vi "Add TypeDef to Cluster.vi"(5 "isArray (F)":bool, 7 "TypeDef path":path, 8 "error in (no error)":errorcluster, 10 "Message Element Name":string, 11 "Owning cluster ref in":refnum<vi>) -> (0 "error out":errorcluster, 2 "Control ref out":refnum<vi>, 3 "Owning cluster ref out":refnum<vi>)   [LabVIEW 2019, in "gRPC Scripting Tools.lvlib"]
uses:
  gRPC Scripting Tools.lvlib
  <vilib>/Utility/miscctls.llb/LVPointTypeDef.ctl
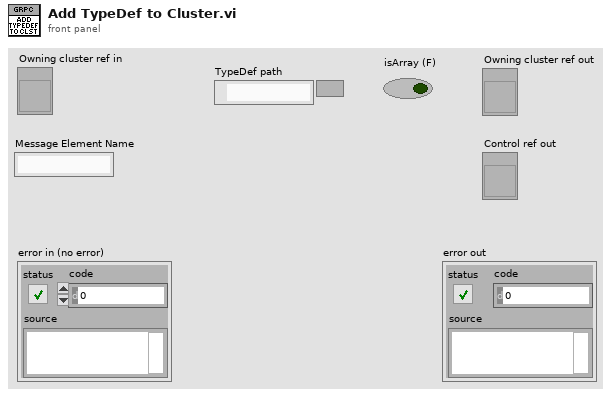
[diagram p1: front panel]
types:
  T1 = typedef "LVPointTypeDef.ctl" = cluster{"Horizontal":i16, "Vertical":i16}
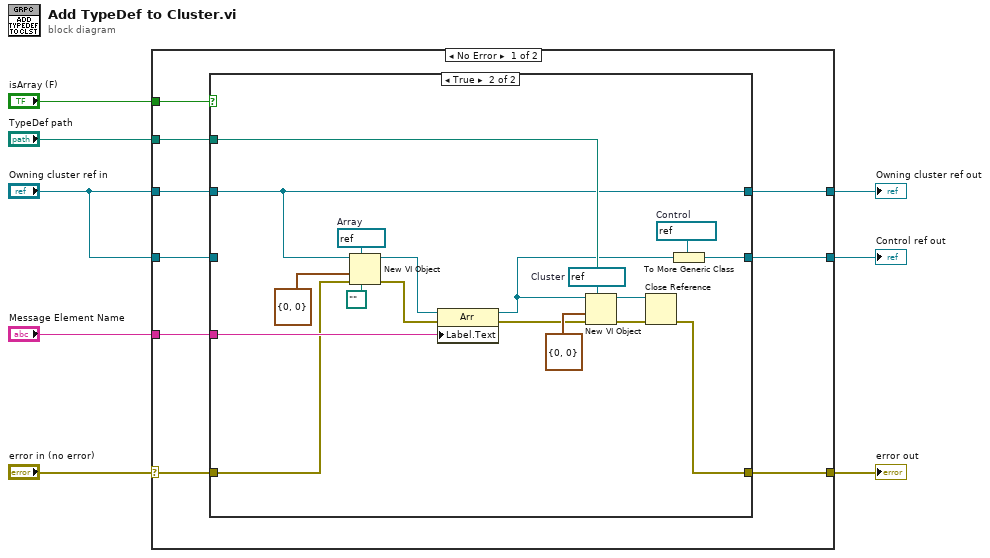
[diagram p0: block diagram]
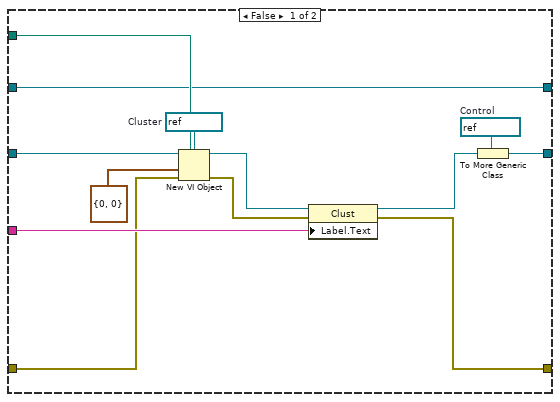
[diagram p2: hidden frame]
diagram:
  n1 = case shown="No Error" "error in (no error)" {
    selector: "error in (no error)" -> [w14 w50]
    tunnel: [w13 w50] -> w8
    tunnel: "TypeDef path" -> [w17 _]
    tunnel: "Owning cluster ref in" -> [w16 _]
    tunnel: "Message Element Name" -> [w15 _]
    tunnel: [w12 _] -> w1
    tunnel: "Owning cluster ref in" -> [w10 w49]
    tunnel: [w9 w49] -> w3
    tunnel: "isArray (F)" -> [w11 _]
    frame No Error {
      n2 = case shown="True" w11 {
        tunnel: w17 -> [w28 w41]
        tunnel: w16 -> [w27 _]
        tunnel: w15 -> [w26 w45]
        tunnel: w14 -> [w23 w36]
        tunnel: [w22 w34] -> w13
        tunnel: [w18 w37] -> w12
        tunnel: w10 -> [w21 w40]
        tunnel: [w21 w40] -> w9
        frame False {
          w20 = refnum<vi> refnum  # Control
          w24 = refnum<vi> refnum  # Cluster
          n3 = New VI Object(vi object class=w24, owner refnum=w27, position/next to=T1 {"Horizontal"=0, "Vertical"=0} ("location"), 6:w28, 8:w23) -> (object refnum=w25:refnum<vi>, 0:w29:errorcluster)  [unwired: 3 in]
          n4 = property class="Clust"(reference=w25, error in=w29, "Label.Text"=w26) -> (reference out=w19:refnum<vi>, error out=w22:errorcluster)
          n5 = To More Generic Class(target class=w20, reference=w19) -> (generic class reference=w18:refnum<vi>)
        }
        frame True {
          w38 = refnum<vi> refnum  # Control
          w43 = refnum<vi> refnum  # Cluster
          w46 = refnum<vi> refnum  # Array
          n6 = New VI Object(vi object class=w46, owner refnum=w40, position/next to=T1 {"Horizontal"=0, "Vertical"=0} ("location"), 6:path "" ("path"), 8:w36) -> (object refnum=w47:refnum<vi>, 0:w48:errorcluster)  [unwired: 3 in]
          n7 = property class="Arr"(reference=w47, error in=w48, "Label.Text"=w45) -> (reference out=w39:refnum<vi>, error out=w42:errorcluster)
          n8 = New VI Object(vi object class=w43, owner refnum=w39, position/next to=T1 {"Horizontal"=0, "Vertical"=0} ("location"), 6:w41, 8:w42) -> (object refnum=w33:refnum<vi>, 0:w35:errorcluster)  [unwired: 3 in]
          n9 = Close Reference(reference=w33, error in (no error)=w35) -> (error out=w34:errorcluster)
          n10 = To More Generic Class(target class=w38, reference=w39) -> (generic class reference=w37:refnum<vi>)
        }
      }
    }
    frame Error {
    }
  }
  "error out" <- w8
  "Owning cluster ref out" <- w3
  "Control ref out" <- w1
